vi "Configure Log Session.vi"(8 "error in":errorcluster, 9 "Path":path, 10 "Ref Name":string, 11 "Configurable Device in":refnum<class "Configurable Device.lvclass">) -> (0 "error out":errorcluster, 3 "Configurable Device out":refnum<class "Configurable Device.lvclass">)   [LabVIEW 2016, in "Configurable Device.lvclass"]
uses:
  Configurable Device.lvclass
  <vilib>/MSR Consulting, LLC/General Reuse/Session APIs/Session Log/System Log.lvclass
  C:/Program Files (x86)/National Instruments/LabVIEW 2016/vi.lib/MSR Consulting, LLC/General Reuse/Session APIs/_Session Fwk/Session - Root.lvclass
  <vilib>/MSR Consulting, LLC/General Reuse/Session APIs/Session Log/System Log.lvclass/System Log.ctl
  Configurable Device.lvclass/Configurable Device.ctl
  <vilib>/MSR Consulting, LLC/General Reuse/Session APIs/Session Log/Accessors/Write Main Path.vi
  <vilib>/MSR Consulting, LLC/General Reuse/Session APIs/_Session Fwk/Session - Root.lvclass
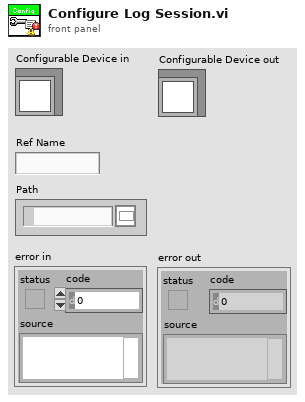
[diagram p1: front panel]
types:
  T1 = typedef "Session - Root.lvclass/Session Handle.ctl" = refnum<data-value>
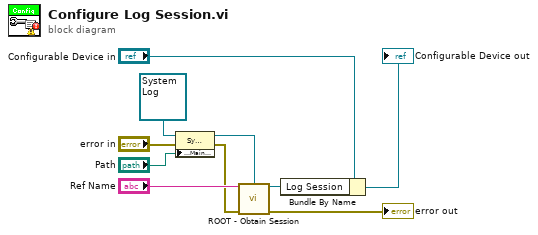
[diagram p0: block diagram]
diagram:
  n1 = property class="Sys Log"(reference=refnum<class "System Log.lvclass"> refnum ("Sys Log"), error in="error in", "Accessors:Main Path"="Path") -> (reference out=w7:refnum<class "System Log.lvclass">, error out=w5:errorcluster)
  n2 = call <vilib>:"ROOT - Obtain Session.vi"("Session Name ()"="Ref Name", "OBJ - Session"=w7, "error in (no error)"=w5) -> ("Session Handle"=w1:T1, "error out"=→"error out":errorcluster)  [unwired: 10 in, 1 out]
  n3 = Bundle By Name(cluster="Configurable Device in", "Log Session"=w1) -> (→"Configurable Device out":refnum<class "Configurable Device.lvclass">)
